vi "FGV_Channel_Cluster.vi"(8 "error in":errorcluster, 10 "Action":T2, 11 "Channel_Cluster_Array IN":T1 {"FW 2" items=["000XX00", "000XX01", "000XX02", "000XX03", "000XX04"]; "FW 1" items=["000XX00", "000XX01", "000XX02", "000XX03", "000XX04"]; "Exposure time" min=0.0 max=5.0 step=0.01; "Power" max=100 step=1}) -> (0 "error out":errorcluster, 3 "Channel_Cluster_Array OUT":T1 {"FW 2" items=["000XX00", "000XX01", "000XX02", "000XX03", "000XX04"]; "FW 1" items=["000XX00", "000XX01", "000XX02", "000XX03", "000XX04"]; "Exposure time" min=0.0 max=5.0 step=0.01; "Power" max=100 step=1})   [LabVIEW 2025]
doc: "Functional Global Variable:\n- Write the value into the memory \nor\n- Read the value from the memory"
uses:
  TypeDef_FGV.ctl
  TypeDef_Array_ChannelCluster.ctl
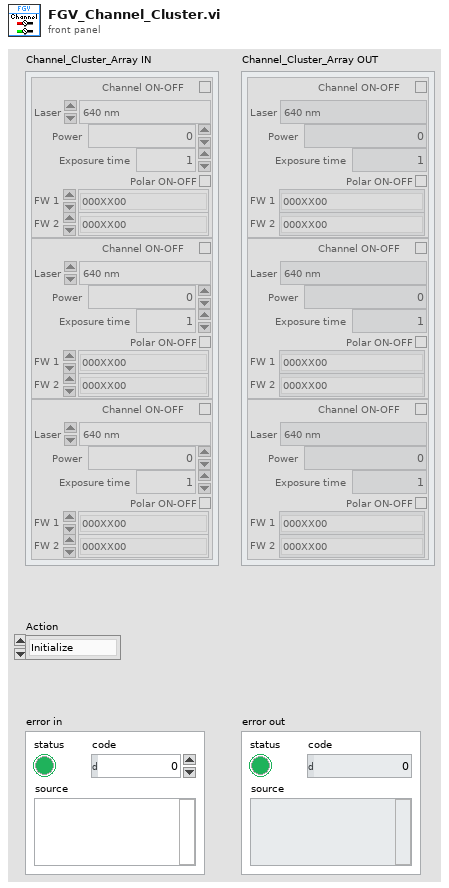
[diagram p1: front panel]
types:
  T1 = typedef "TypeDef_Array_ChannelCluster.ctl" = cluster{"Laser":enum16{"640 nm", "561 nm"}, "Power":u8, "Exposure time":dbl, "Channel ON-OFF":bool, "Polar ON-OFF":bool, "FW 1":u16, "FW 2":u16}[]
  T2 = typedef "TypeDef_FGV.ctl" = enum16{"Initialize", "Write", "Read", "Read_File", "Write_to_File"}
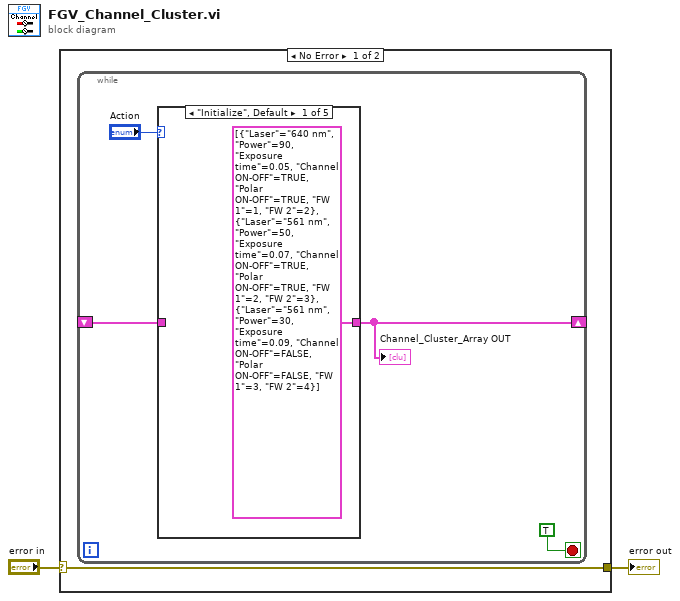
[diagram p0: block diagram]
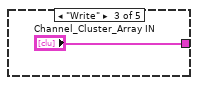
[diagram p3: hidden frame]
diagram:
  n1 = case shown="No Error" "error in" {
    selector: "error in" -> [w3 w13]
    tunnel: [w3 w13] -> w1
    frame No Error {
      n2 = while {
        shift-right: [w4] -> _
        shift-left: _ -> [w5]
        stop <- TRUE stop-if-true
        n3 = case shown="\"Initialize\", Default" "Action" {
          tunnel: w5 -> [_ w9 _ w11 w12]
          tunnel: [T1 [{"Laser"=enum."640 nm", "Power"=90, "Exposure time"=0.05, "Channel ON-OFF"=TRUE, "Polar ON-OFF"=TRUE, "FW 1"=1, "FW 2"=2}, {"Laser"=enum."561 nm", "Power"=50, "Exposure time"=0.07, "Channel ON-OFF"=TRUE, "Polar ON-OFF"=TRUE, "FW 1"=2, "FW 2"=3}, {"Laser"=enum."561 nm", "Power"=30, "Exposure time"=0.09, "Channel ON-OFF"=FALSE, "Polar ON-OFF"=FALSE, "FW 1"=3, "FW 2"=4}] ("Channel_Cluster_Array OUT") w9 "Channel_Cluster_Array IN" w11 w12] -> w4
          frame "Initialize", Default {
          }
          frame "Read" {
          }
          frame "Write" {
          }
          frame "Read_File" {
            # "A FAIRE"
          }
          frame "Write_to_File" {
            # "A Faire"
          }
        }
        "Channel_Cluster_Array OUT" <- w4
      }
    }
    frame Error {
    }
  }
  "error out" <- w1
